vi "EMBALLAGE_BDD_typeProduit_GPAO.vi"(0 "NOS_ARTICLE(%)":string, 1 "Famille":string, 3 "affiche code barre client":string, 4 "date":string, 5 "error in (no error)":errorcluster, 6 "indice_produit":string, 7 "clc_designation":string, 9 "Mélange_lots_possible":string, 10 "longeur_No_série":string, 11 "SUFFIXE":string, 12 "Code_barre_fixe":string, 13 "Code_barre_fixe_fin":string) -> (14 "Tableau":string[][](array[string]), 19 "error out":errorcluster)   [LabVIEW 2020]
uses:
  Modules/FS/60_FS_Controles/60_FS_SetGet.ctl
  <vilib>/addons/database/Connection.llb/DB Tools Open Connec (Path).vi
  <vilib>/addons/database/Connection.llb/Conn Execute.vi
  <vilib>/addons/database/Recordset.llb/Rec Fetch Recordset Data (R).vi
  <vilib>/addons/database/Recordset.llb/Rec Destroy - Connection.vi
  <vilib>/addons/database/NI_Database_API.lvlib
panel:
  out "sep_code_barre":string
  out "champ_Code_Barre":string
  out "champ_Indice":string
  out "sep_code_barre_indice":string
  out "données":string[][](array[string])
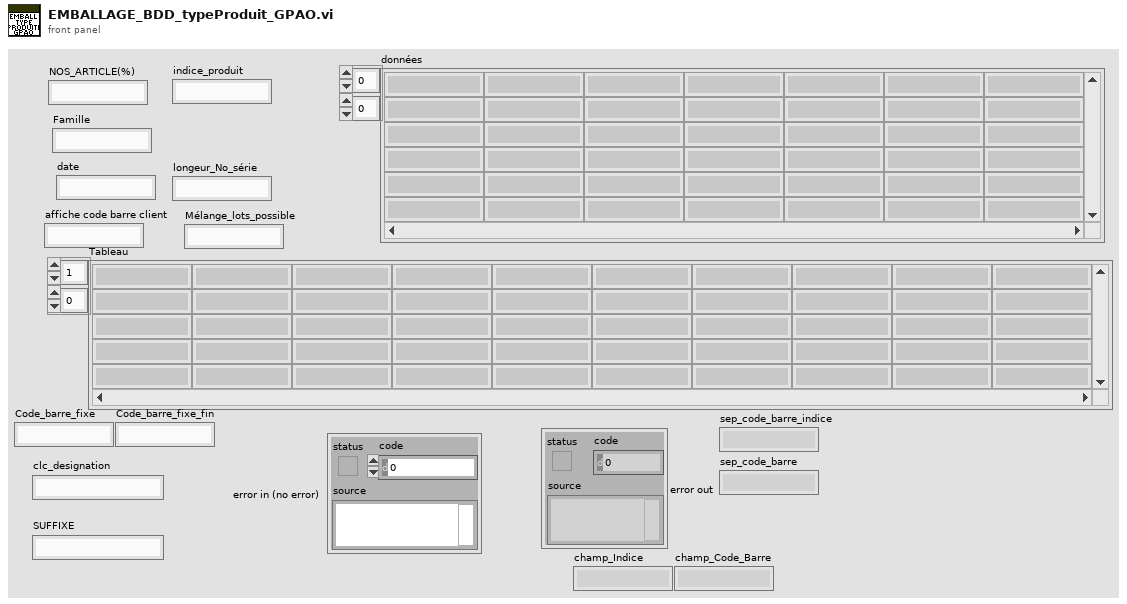
[diagram p1: front panel]
types:
  T1 = typedef "60_FS_SetGet.ctl" = enum16{"set", "get"}
  T2 = typedef "60_FS_CLT_Chemins.ctl" = cluster{"Racine_local":path, "Racine_reseau":path, "Racine_Support_Application":path, "Fichier_Journalisation":path, "Connexion_BDD_VSX":path, "Connexion_BDD_PLZ":path}
  T3 = typedef "NI_Database_API.lvlib/Conn ObjectReference.ctl" = refnum<k1>
  T4 = typedef "NI_Database_API.lvlib/Rec ObjectReference.ctl" = refnum<k1>
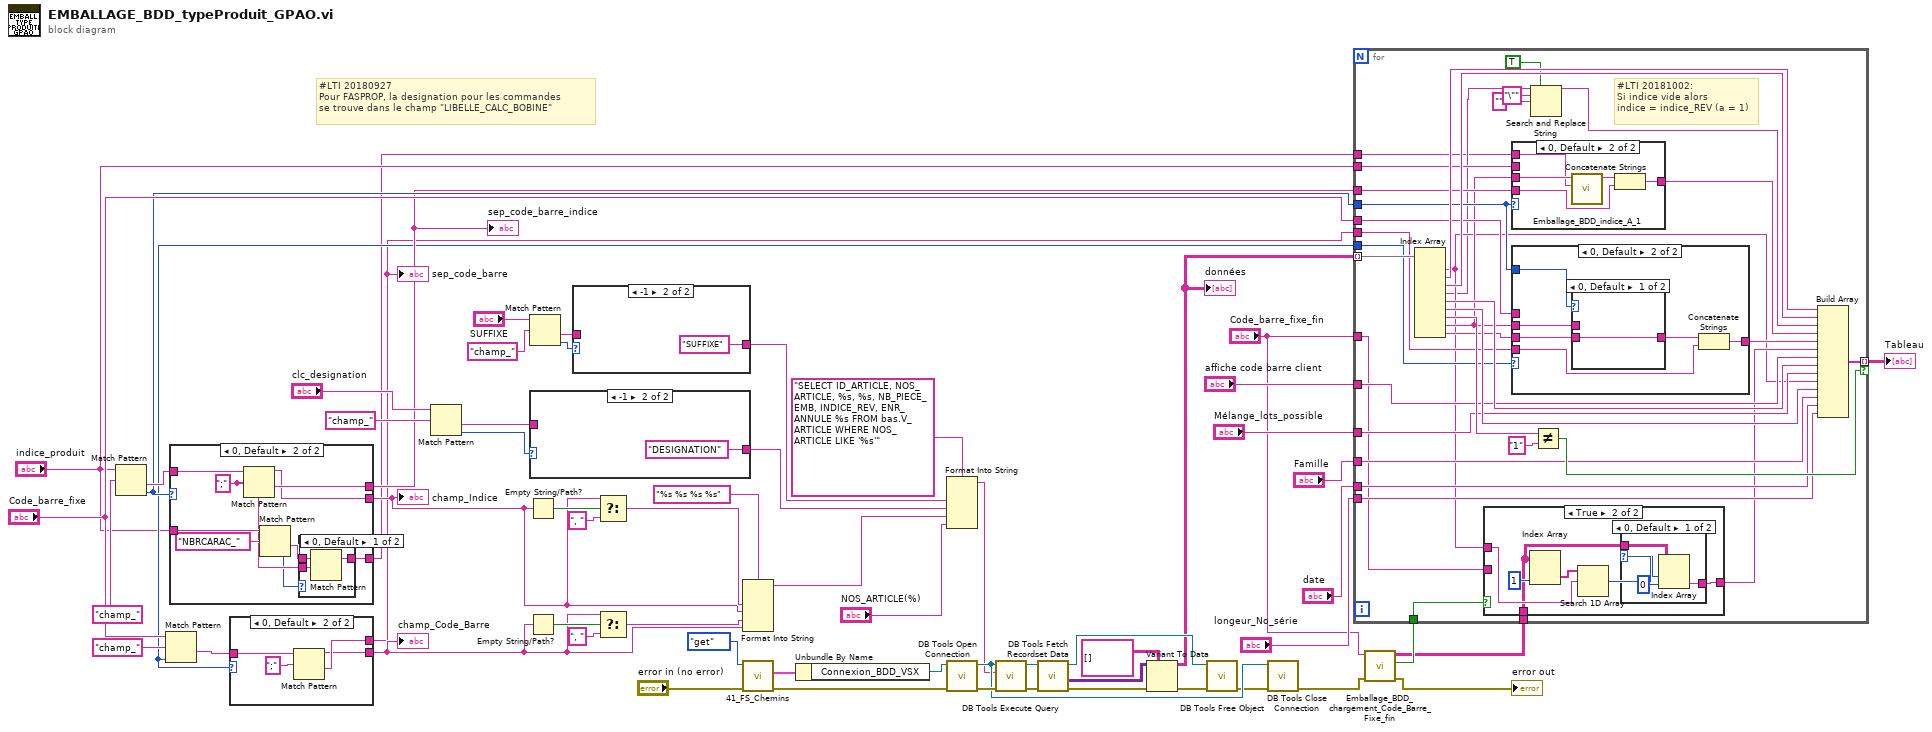
[diagram p0: block diagram]
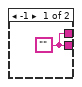
[diagram p2: hidden frame]
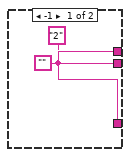
[diagram p3: hidden frame]
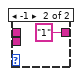
[diagram p4: hidden frame]
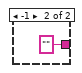
[diagram p8: hidden frame]
diagram:
  # "#LTI 20180927\nPour FASPROP, la designation pour les commandes \nse trouve dans le champ \"LIBELLE_CALC_BOBINE\""
  n1 = Match Pattern(string="indice_produit", regular expression="champ_" ("expression régulière")) -> (after substring=w31:string, offset past match=w13:i32)  [unwired: 1 in, 2 out]
  n2 = Match Pattern(string="Code_barre_fixe", regular expression="champ_" ("expression régulière")) -> (after substring=w24:string, offset past match=w11:i32)  [unwired: 1 in, 2 out]
  n3 = case shown="0, Default" w13 {
    tunnel: w31 -> [_ w72]
    tunnel: [w63 w71] -> w12
    tunnel: [w63 w70] -> w18
    tunnel: "indice_produit" -> [_ w69]
    tunnel: ["2" ("indice_produit") w65] -> w1
    frame -1 {
      w63 = ""
    }
    frame 0, Default {
      w66 = ";" ("expression régulière")
      n4 = Match Pattern(string=w72, regular expression=w66) -> (before substring=w70:string, after substring=w71:string)  [unwired: 1 in, 2 out]
      n5 = Match Pattern(string=w69, regular expression="NBRCARAC_" ("expression régulière")) -> (after substring=w67:string, offset past match=w64:i32)  [unwired: 1 in, 2 out]
      n6 = case shown="0, Default" w64 {
        tunnel: w67 -> [w75 _]
        tunnel: w66 -> [w74 _]
        tunnel: [w73 "1" ("indice_produit")] -> w65
        frame 0, Default {
          n7 = Match Pattern(string=w75, regular expression=w74) -> (before substring=w73:string)  [unwired: 1 in, 3 out]
        }
        frame -1 {
        }
      }
    }
  }
  "sep_code_barre_indice" <- w12
  "champ_Indice" <- w18
  n8 = case shown="0, Default" w11 {
    tunnel: w24 -> [_ w81]
    tunnel: [w77 w79] -> w10
    tunnel: [w77 w78] -> w14
    frame -1 {
      w77 = ""
    }
    frame 0, Default {
      n9 = Match Pattern(string=w81, regular expression=";" ("expression régulière")) -> (before substring=w78:string, after substring=w79:string)  [unwired: 1 in, 2 out]
    }
  }
  "champ_Code_Barre" <- w14
  "sep_code_barre" <- w10
  n10 = Match Pattern(string="clc_designation", regular expression="champ_" ("expression régulière")) -> (after substring=w38:string, offset past match=w41:i32)  [unwired: 1 in, 2 out]
  n11 = Empty String/Path?(string/path=w18) -> (empty?=w21:bool)
  n12 = Empty String/Path?(string/path=w14) -> (empty?=w17:bool)
  n13 = Match Pattern(string="SUFFIXE", regular expression="champ_" ("expression régulière")) -> (after substring=w35:string, offset past match=w34:i32)  [unwired: 1 in, 2 out]
  n14 = case shown="-1" w41 {
    tunnel: [w82 "DESIGNATION"] -> w39
    tunnel: w38 -> [w82 _]
    frame 0, Default {
    }
    frame -1 {
    }
  }
  n15 = case shown="-1" w34 {
    tunnel: [w84 "SUFFIXE"] -> w33
    tunnel: w35 -> [w84 _]
    frame 0, Default {
    }
    frame -1 {
    }
  }
  n16 = Select(t=w18, s=w21, f=", " ("cas faux")) -> (s? t:f=w20:string)
  n17 = Select(t=w14, s=w17, f=", " ("cas faux")) -> (s? t:f=w15:string)
  n18 = Format Into String(format string="%s %s %s %s" ("chaîne de format"), w20, w18, w15, w14) -> (resulting string=w8:string)  [unwired: 2 in, 1 out]
  n19 = call "41_FS_Chemins.vi"("error in (no error)"="error in (no error)", "SetGet"=60_FS_SetGet."get") -> ("error out"=w50:errorcluster, "CLT_Chemins_out"=w49:T2)  [unwired: 8 in]
  n20 = Unbundle By Name(w49) -> ("Connexion_BDD_VSX"=w59:path)
  n21 = Format Into String(format string="SELECT ID_ARTICLE, NOS_ARTICLE, %s, %s, NB_PIECE_EMB, INDICE_REV, ENR_ANNULE %s FROM bas.V_ARTICLE WHERE NOS_ARTICLE LIKE '%s'" ("SQL query"), w33, w39, w8, "NOS_ARTICLE(%)") -> (resulting string=w46:string)  [unwired: 2 in, 1 out]
  n22 = call-poly <vilib>:"DB Tools Open Connection.vi"("error in (no error)"=w50, "connection information"=w59) -> ("error out"=w61:errorcluster, "connection reference"=w60:T3)  [unwired: 6 in]
  n23 = call-poly <vilib>:"DB Tools Execute Query.vi"("error in (no error)"=w61, "SQL query"=w46, "connection reference"=w60) -> ("error out"=w51:errorcluster, "recordset reference"=w52:T4)  [unwired: 5 in]
  n24 = call-poly <vilib>:"DB Tools Fetch Recordset Data.vi"("error in (no error)"=w51, "recordset reference"=w52) -> ("error out"=w54:errorcluster, "recordset data"=w53:variant[][], "recordset reference out"=w57:T4)  [unwired: 3 in]
  n25 = Variant To Data(error in=w54, type=string[][] [] ("Chaînes []"), Variant=w53) -> (data=w45:string[][], error out=w56:errorcluster)
  "données" <- w45
  n26 = call-poly <vilib>:"DB Tools Free Object.vi"("error in (no error)"=w56, "recordset reference"=w57) -> ("error out"=w58:errorcluster)  [unwired: 8 in, 1 out]
  n27 = call <vilib>:"DB Tools Close Connection.vi"("error in (no error)"=w58, "connection reference"=w60) -> ("error out"=w7:errorcluster)  [unwired: 5 in]
  n28 = call "Emballage_BDD_chargement_Code_Barre_Fixe_fin.vi"("Error in"=w7, "code_barre_fixe_fin"="Code_barre_fixe_fin") -> ("Error out"=→"error out":errorcluster, "code_barre_fixe_fichier?"=w4:bool, "tbl_Autre_Article"=w3:string[][])  [unwired: 7 in]
  n29 = for {
    tunnel: w45 -> [w120] mode=indexing
    tunnel: [w116] -> w44 mode=indexing if=w113
    tunnel: "indice_produit" -> [w106]
    tunnel: "Code_barre_fixe" -> [w102]
    tunnel: "affiche code barre client" -> [w111]
    tunnel: "Mélange_lots_possible" -> [w110]
    tunnel: "Famille" -> [w109]
    tunnel: "date" -> [w108]
    tunnel: "longeur_No_série" -> [w107]
    tunnel: "Code_barre_fixe_fin" -> [w95]
    tunnel: w13 -> [w99]
    tunnel: w12 -> [w104]
    tunnel: w11 -> [w101]
    tunnel: w10 -> [w100]
    tunnel: w4 -> [w96]
    tunnel: w3 -> [w93]
    tunnel: w1 -> [w86]
    # "#LTI 20181002:\nSi indice vide alors\nindice = indice_REV (a = 1)"
    n30 = Index Array(array=w120) -> (element #1=w92:string, element #2=w119:string, element #3=w118:string, element #4=w90:string, element #5=w117:string, element #6=w112:string, element #7=w115:string, element #8=w98:string, element #9=w97:string)  [unwired: 9 in]
    n31 = case shown="True" w96 {
      tunnel: w95 -> [w121 _]
      tunnel: [w121 w123] -> w94
      tunnel: w93 -> [_ w122]
      tunnel: w92 -> [_ w125]
      frame False {
      }
      frame True {
        n32 = Index Array(array=w122, index (col)=1 ("indice (col)")) -> (element=w126:string[])  [unwired: 1 in]
        n33 = Search 1D Array(1D array=w126, element=w125) -> (index of element=w124:i32)  [unwired: 1 in]
        n34 = case shown="0, Default" w124 {
          selector: w124 -> [w129 _]
          tunnel: [w128 "" ("Code_barre_fixe_fin")] -> w123
          tunnel: w122 -> [w131 _]
          frame 0, Default {
            n35 = Index Array(array=w131, index (row)=w129, index (col)=0 ("indice désactivé (col)")) -> (element=w128:string)
          }
          frame -1 {
          }
        }
      }
    }
    n36 = case shown="0, Default" w99 {
      tunnel: w106 -> [w142 _]
      tunnel: [w142 w145] -> w105
      tunnel: w98 -> [_ w147]
      tunnel: w104 -> [_ w144]
      tunnel: w86 -> [_ w143]
      frame -1 {
      }
      frame 0, Default {
        n37 = call "Emballage_BDD_indice_A_1.vi"("NbrDeCar."=w143, "indiceLettre"=w147) -> ("indiceAttenduNum"=w146:string)  [unwired: 9 in]
        n38 = Concatenate Strings(w146, w144) -> (w145:string)
      }
    }
    n39 = case shown="0, Default" w101 {
      tunnel: w102 -> [w133 _]
      tunnel: [w133 w139] -> w103
      tunnel: w100 -> [_ w138]
      tunnel: w99 -> [_ w137]
      tunnel: w98 -> [_ w135]
      tunnel: w97 -> [_ w134]
      frame -1 {
      }
      frame 0, Default {
        n40 = case shown="0, Default" w137 {
          tunnel: [w140 w141] -> w136
          tunnel: w135 -> [_ w141]
          tunnel: w134 -> [w140 _]
          frame 0, Default {
          }
          frame -1 {
          }
        }
        n41 = Concatenate Strings(w136, w138) -> (w139:string)
      }
    }
    n42 = Search and Replace String(replace all?=TRUE ("tout remplacer ? (F)"), input string=w90, search string="\"" ("chaîne recherchée"), replace string="" ("chaîne de remplacement (\"\")")) -> (result string=w91:string)  [unwired: 4 in, 3 out]
    n43 = Not Equal?(x=w115, y="1") -> (x != y?=w113:bool)
    n44 = Build Array(w119, w118, w91, w105, w103, w94, w111, w117, w110, w92, w112, w109, w108, w107) -> (w116:string[])
  }
  "Tableau" <- w44
